vi "WaitForListener.vi"(0 "Socket Listener in":refnum<class "Socket Communication.lvclass">, 5 "error in (no error)":errorcluster, 9 "Timeout (ms)":i32=100) -> (14 "Socket Listener out":refnum<class "Socket Communication.lvclass">, 19 "error out":errorcluster)   [LabVIEW 2016, in "Socket Communication.lvclass"]
uses:
  Socket Communication.lvclass
  Socket Communication.lvclass/Socket Communication.ctl
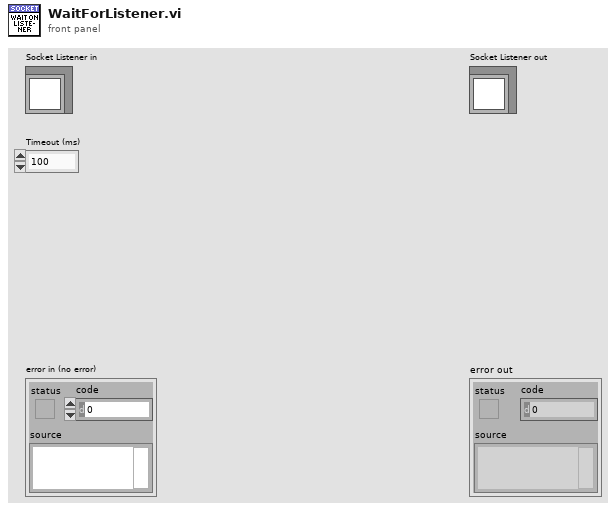
[diagram p1: front panel]
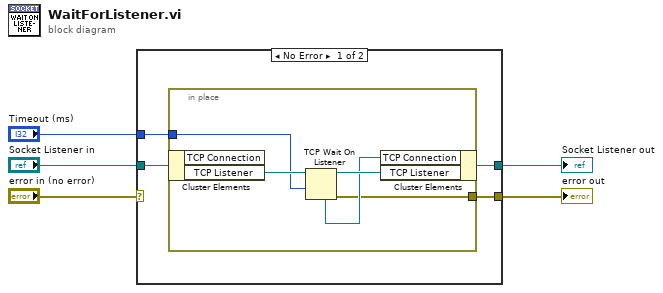
[diagram p0: block diagram]
diagram:
  n1 = case shown="No Error" "error in (no error)" {
    selector: "error in (no error)" -> [_ w16]
    tunnel: [w7 w16] -> w4
    tunnel: [w8 w15] -> w2
    tunnel: "Socket Listener in" -> [w9 w15]
    tunnel: "Timeout (ms)" -> [w6 _]
    frame No Error {
      n2 = in-place {
        in-place-border: [w11] -> w7
        in-place-border: w6 -> [w10]
        n3 = in-place-cluster #1(w9) -> ("TCP Listener"=w14:refnum<k5>)  [unwired: 1 out]
        n4 = TCP Wait On Listener(9:w10, 11:w14) -> (0:w11:errorcluster, 3:w13:refnum<k5>, 4:w12:refnum<k5>)  [unwired: 2 in, 2 out]
        n5 = in-place-cluster #1("TCP Connection"=w12, "TCP Listener"=w13) -> (w8:refnum<class "Socket Communication.lvclass">)
      }
    }
    frame Error {
    }
  }
  "error out" <- w4
  "Socket Listener out" <- w2
